vi "PR Set Trigger Source.vi"(0 "TriggerSource":i32) -> ()   [LabVIEW 2022 SP3, in "BS6006PRPLUS.lvlib"]
doc: "The function sets the trigger source of pulser/receiver.\n\nextern \"C\" BS6006PRPLUS_API void __cdecl PR_SetTriggerSource(int TriggerSource);"
uses:
  BS6006PRPLUS.lvlib
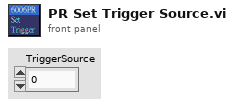
[diagram p1: front panel]
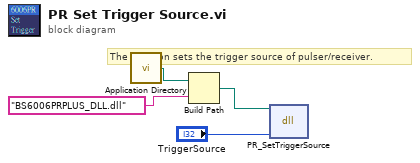
[diagram p0: block diagram]
diagram:
  # "The function sets the trigger source of pulser/receiver."
  n1 = call <vilib>:"Application Directory.vi"() -> ("Application Directory"=w3:path)
  n2 = Build Path(base path=w3, name or relative path="BS6006PRPLUS_DLL.dll") -> (appended path=w1:path)
  n3 = dll-call lib="E:/Broadsound_Program/PulserReceiver/6006PR PLUS/API/DLL/LabVIEW 15/VIs/BS6006PRPLUS_DLL.dll" fn="PR_SetTriggerSource"(path in=w1, "TriggerSource"="TriggerSource") -> ()  [unwired: 4 in, 2 out]
